vi "64-bit Number to SGL Complex.vi"(7 "Input":u64) -> (8 "Complex Number":T1)   [LabVIEW 2011]
uses:
  <vilib>/rvi/FXPMathLib/FxpInterpret/XNode/nifxpmath_Interpret.xnode
types:
  T1 = cluster{"xk_im":fxp<+,32,32>, "xk_re":fxp<+,32,32>}
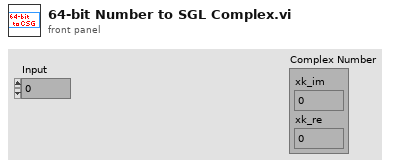
[diagram p1: front panel]
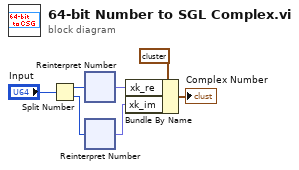
[diagram p0: block diagram]
diagram:
  n1 = Split Number(x="Input") -> (hi(x)=w6:u32, lo(x)=w4:u32)
  n2 = xnode "Reinterpret Number"("x"=w6) -> ("y"=w5:fxp<+,32,32>)
  n3 = xnode "Reinterpret Number"("x"=w4) -> ("y"=w3:fxp<+,32,32>)
  n4 = Bundle By Name(cluster=T1 {"xk_im"=0.0, "xk_re"=0.0} ("FFT Output"), "xk_re"=w5, "xk_im"=w3) -> (→"Complex Number":T1)
